vi "Zero Adjust MFC.vi"(8 "Error In":errorcluster, 10 "Channel (0)":i32, 11 "VISA resource name":refnum<visa-resource-name>) -> (0 "Error Out":errorcluster, 1 "MFC Offset":dbl[unit], 3 "dup VISA resource name":refnum<visa-resource-name>)   [LabVIEW 2016, in "MGC647C.lvlib"]
doc: "Zero adjust MFC of a channel."
uses:
  MGC647C.lvlib
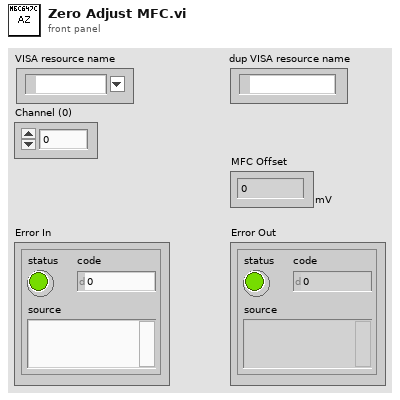
[diagram p1: front panel]
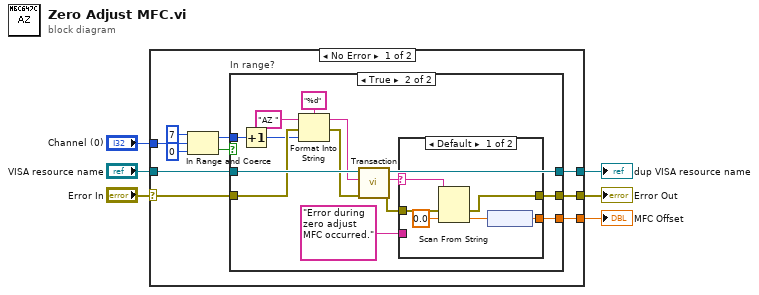
[diagram p0: block diagram]
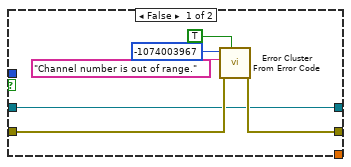
[diagram p2: hidden frame]
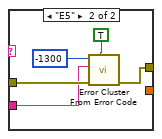
[diagram p3: hidden frame]
diagram:
  n1 = case shown="No Error" "Error In" {
    selector: "Error In" -> [w13 w49]
    tunnel: "VISA resource name" -> [w16 w48]
    tunnel: [w15 w48] -> w5
    tunnel: [w14 w49] -> w4
    tunnel: "Channel (0)" -> [w10 _]
    tunnel: [w7 _] -> w1
    frame No Error {
      n2 = In Range and Coerce(upper limit=7, x=w10, lower limit=0) -> (coerced(x)=w9:i32, In Range?=w8:bool)
      n3 = case "In range?" shown="True" w8 {
        tunnel: w16 -> [w20 w36]
        tunnel: [w20 w35] -> w15
        tunnel: [w21 w31] -> w14
        tunnel: w13 -> [w22 w34]
        tunnel: w9 -> [_ w30]
        tunnel: [_ w25] -> w7
        frame False {
          n4 = call <vilib>:"Error Cluster From Error Code.vi"("show call chain? (False)"=TRUE, "error in (no error)"=w22, "error message (\"\")"="Channel number is out of range." ("error message (\"\")"), "error code (0)"=-1074003967) -> ("error out"=w21:errorcluster)  [unwired: 5 in]
        }
        frame True {
          n5 = Increment(x=w30) -> (x+1=w29:i32)
          n6 = Format Into String(format string="%d", initial string="AZ " ("string (\"\")"), error in=w34, w29) -> (resulting string=w27:string, error out=w33:errorcluster)
          n7 = call "Transaction.vi"("Error In"=w33, "Command"=w27, "VISA resource name"=w36) -> ("Error Out"=w32:errorcluster, "Response"=w24:string, "dup VISA resource name"=w35:refnum<visa-resource-name>)  [unwired: 6 in]
          n8 = case shown="Default" w24 {
            selector: w24 -> [w37 _]
            tunnel: w32 -> [w42 w46]
            tunnel: [w41 w47] -> w31
            tunnel: [w38 _] -> w25
            tunnel: "Error during zero adjust MFC occurred." ("error source (\" \")") -> [_ w44]
            frame Default {
              n9 = Scan From String(input string=w37, error in=w42, default 1=0.0 ("default value 1")) -> (error out=w41:errorcluster, output 1=w39:dbl)  [unwired: 2 in, 2 out]
              n10 = node(w39) -> (w38:dbl[unit])
            }
            frame "E5" {
              n11 = call <vilib>:"Error Cluster From Error Code.vi"("show call chain? (False)"=TRUE, "error in (no error)"=w46, "error message (\"\")"=w44, "error code (0)"=-1300 ("error code (no error:0)")) -> ("error out"=w47:errorcluster)  [unwired: 5 in]
            }
          }
        }
      }
    }
    frame Error {
    }
  }
  "dup VISA resource name" <- w5
  "Error Out" <- w4
  "MFC Offset" <- w1
